vi "Do.vi"(8 "error in (no error)":errorcluster, 10 "Actor in":refnum<class "Actor.lvclass">, 11 "ppanel_change_hydraharp_settings Msg":refnum<class "ppanel_change_hydraharp_settings Msg.lvclass">) -> (0 "error out":errorcluster, 2 "Actor out":refnum<class "Actor.lvclass">)   [LabVIEW 2015, in "ppanel_change_hydraharp_settings Msg.lvclass"]
doc: "This VI delivers the message to the actor by calling the appropriate method(s) on the actor."
uses:
  ppanel_change_hydraharp_settings Msg.lvclass
  <vilib>/ActorFramework/Actor/Actor.lvclass
  picoharp_panel/picoharp_panel.lvclass
  ppanel_change_hydraharp_settings Msg.lvclass/ppanel_change_hydraharp_settings Msg.ctl
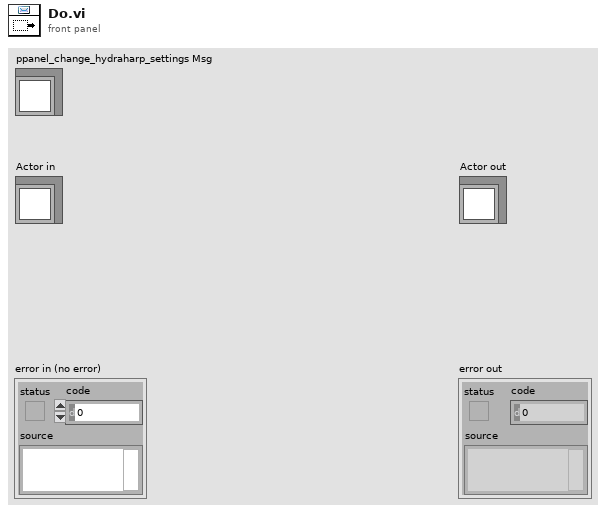
[diagram p1: front panel]
types:
  T1 = typedef "hpanel_hydraharp_settings.ctl" = cluster{"Sync Settings":T2, "CH 1":T4, "CH 2":T4, "CH 3":T4, "CH 4":T4, "binning":i32, "CH 5":T4, "CH 6":T4, "CH 7":T4, "CH 8":T4}
  T2 = typedef "hpanel_sync_settings.ctl" = cluster{"snc_count":i32, "snc_level":i32, "snc_ZeroX":i32, "snc_offs":i32, "sync_div":T3}
  T3 = typedef "hpanel_sync_div.ctl" = enum16{"1", "2", "4", "8"}
  T4 = typedef "hpanel_channel_settings.ctl" = cluster{"ch_counts":i32, "ch_level":i32, "ch_ZeroX":i32, "ch_offs":i32}
  T5 = typedef "hpanel_acq_modes.ctl" = u16
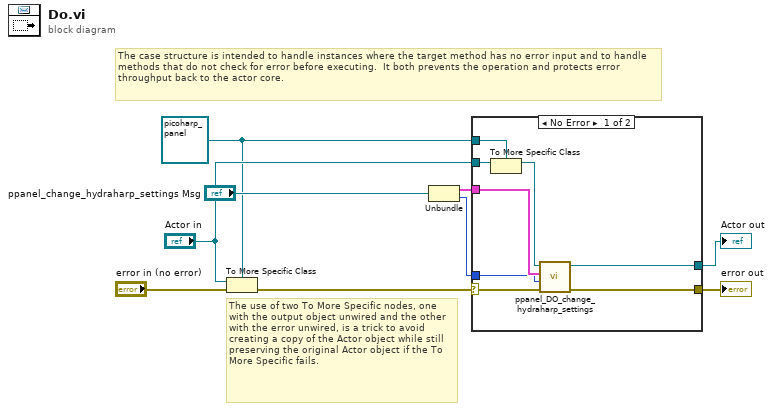
[diagram p0: block diagram]
diagram:
  w3 = refnum<class "picoharp_panel.lvclass"> refnum ("Actor in")
  # "The use of two To More Specific nodes, one with the output object unwired and the other with the error unwired, is a trick to avoid creating a copy of the Actor object while still preserving the original Actor object if the To More Specific fails."
  # "The case structure is intended to handle instances where the target method has no error input and to handle methods that do not check for error before executing.  It both prevents the operation and protects error throughput back to the actor core."
  n1 = To More Specific Class(target class=w3, reference="Actor in", error in="error in (no error)") -> (error out=w7:errorcluster)  [unwired: 1 out]
  n2 = Unbundle("ppanel_change_hydraharp_settings Msg") -> (w2:T1, w1:T5)
  n3 = case shown="No Error" w7 {
    selector: w7 -> [w15 w19]
    tunnel: [w17 w19] -> w6
    tunnel: [w16 w18] -> w5
    tunnel: "Actor in" -> [w14 w18]
    tunnel: w3 -> [w13 _]
    tunnel: w2 -> [w11 _]
    tunnel: w1 -> [w10 _]
    frame No Error {
      n4 = To More Specific Class(target class=w13, reference=w14) -> (specific class reference=w12:refnum<class "picoharp_panel.lvclass">)  [unwired: 1 in, 1 out]
      n5 = call "ppanel_DO_change_hydraharp_settings.vi"("error in (no error)"=w15, "Mode"=w10, "Hydraharp Settings"=w11, "hydraharp_panel in"=w12) -> ("error out"=w17:errorcluster, "hydraharp_panel out"=w16:refnum<class "picoharp_panel.lvclass">)  [unwired: 6 in]
    }
    frame Error {
      # "If type check fails, pass the original object out again."
    }
  }
  "error out" <- w6
  "Actor out" <- w5
